vi "Init Command Panel.vi"(8 "error in (no error)":errorcluster, 10 "VolatusAPI":refnum<class "VolatusAPI.lvclass">, 11 "Command Panel in":refnum<class "Command Panel.lvclass">) -> (0 "error out":errorcluster, 3 "Command Panel out":refnum<class "Command Panel.lvclass">)   [LabVIEW 2020, in "VolatusGUI.lvlib" / "Command Panel.lvclass"]
uses:
  Command Panel.lvclass
  Volatus/VolatusAPI/VolatusAPI.lvclass
  Command Panel.lvclass/Command Panel.ctl
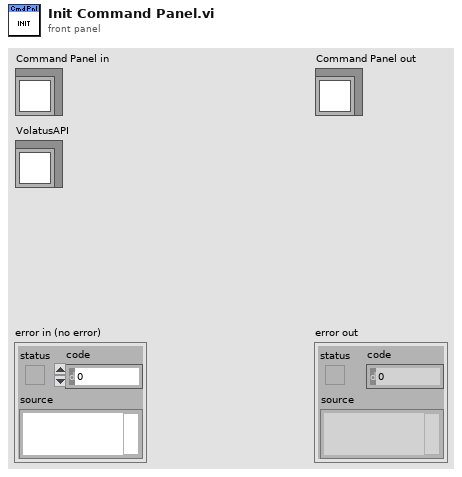
[diagram p1: front panel]
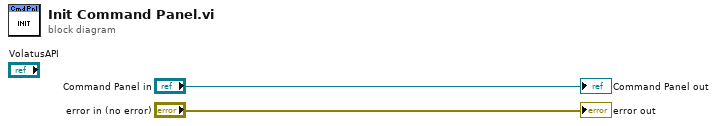
[diagram p0: block diagram]
diagram:
  "error out" <- "error in (no error)"
  "Command Panel out" <- "Command Panel in"
